vi "MainConvertiMisure_OUTPUT.vi"() -> ()   [LabVIEW 2016]
uses:
  <vilib>/Utility/file.llb/Read Delimited Spreadsheet (string).vi
panel:
  out "Array Miure Convertite":dbl[](array[numeric])
  out "Caratteristiche Caricate":string[][](array[string])
  in  "Array Misure Input":dbl[](array[numeric])
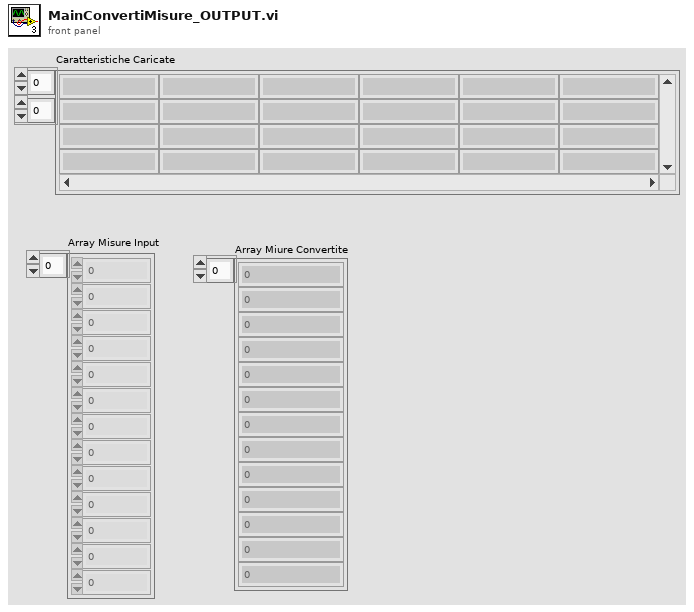
[diagram p1: front panel]
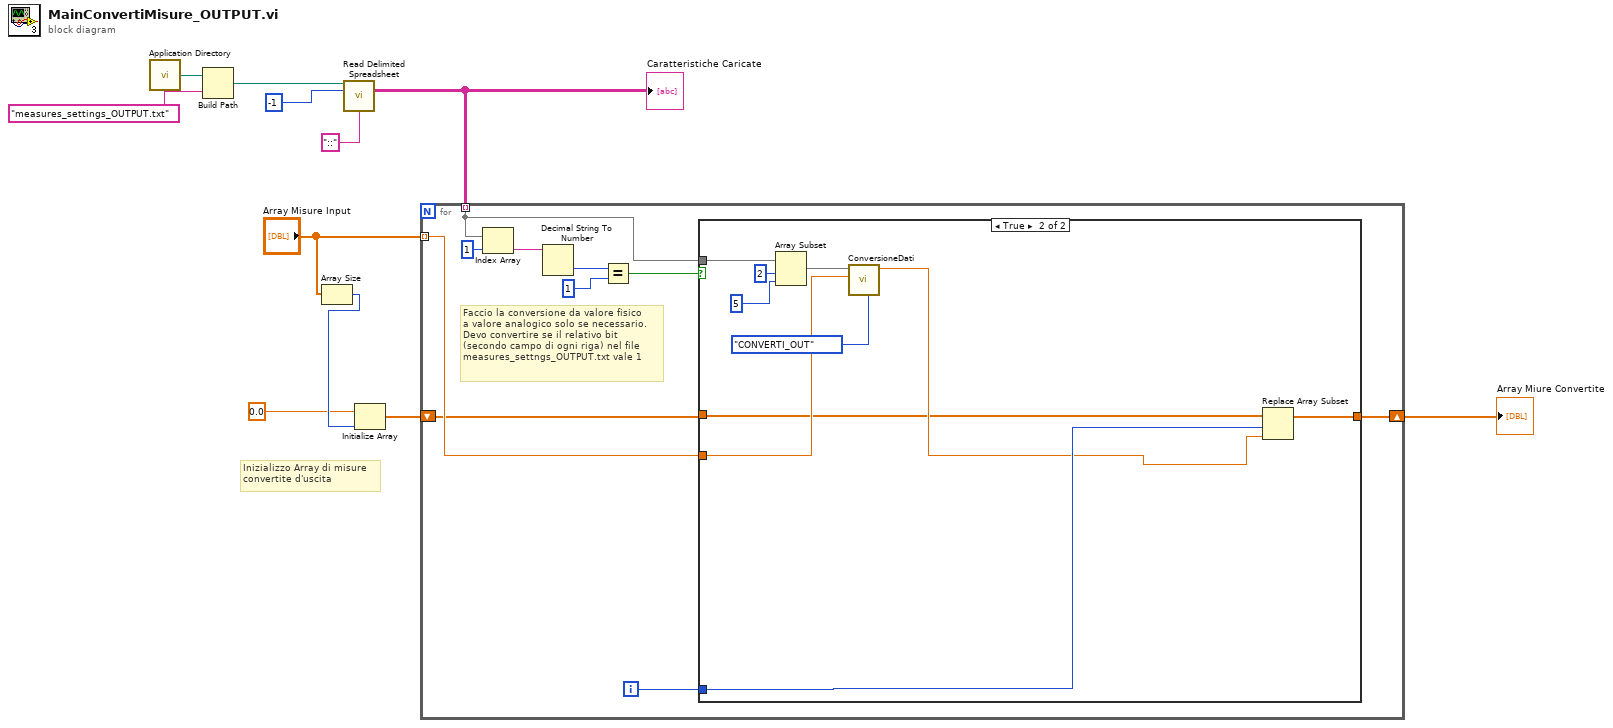
[diagram p0: block diagram]
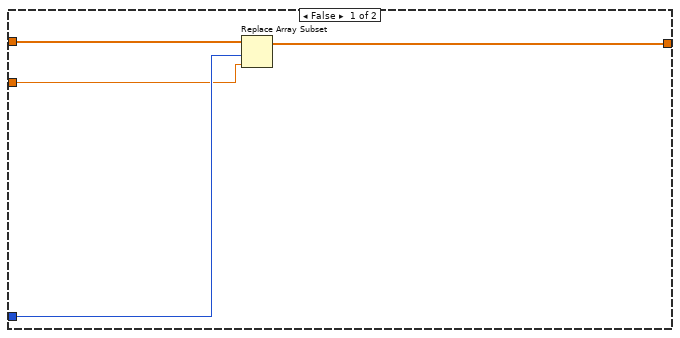
[diagram p2: hidden frame]
diagram:
  # "Inizializzo Array di misure \nconvertite d'uscita"
  n1 = call <vilib>:"Application Directory.vi"() -> ("Application Directory"=w10:path)
  n2 = Build Path(base path=w10, name or relative path="measures_settings_OUTPUT.txt") -> (appended path=w9:path)
  n3 = Array Size(array="Array Misure Input") -> (size(s)=w4:i32)
  n4 = call-poly <vilib>:"Read Delimited Spreadsheet.vi"("file path (dialog if empty)"=w9, "number of rows (all:-1)"=-1, "delimiter (\\t)"="::" ("delimiter (\\t)")) -> ("all rows"=w6:string[][])  [unwired: 7 in, 5 out]
  "Caratteristiche Caricate" <- w6
  n5 = Initialize Array(0.0, w4) -> (w2:dbl[])
  n6 = for {
    tunnel: "Array Misure Input" -> [w16] mode=indexing
    tunnel: w6 -> [w13] mode=indexing
    shift-right: [w14] -> w1
    shift-left: w2 -> [w15]
    i -> [w12]
    # "Faccio la conversione da valore fisico\na valore analogico solo se necessario. \nDevo convertire se il relativo bit \n(secondo campo di ogni riga) nel file \nmeasures_settngs_OUTPUT.txt vale 1"
    n7 = Index Array(array=w13, index=1) -> (element=w20:string)
    n8 = Decimal String To Number(string=w20) -> (number=w19:i32)  [unwired: 2 in, 1 out]
    n9 = Equal?(x=w19, y=1) -> (x = y?=w17:bool)
    n10 = case shown="True" w17 {
      tunnel: w16 -> [w24 w31]
      tunnel: w15 -> [w22 w26]
      tunnel: w12 -> [w25 w35]
      tunnel: [w23 w34] -> w14
      tunnel: w13 -> [_ w33]
      frame False {
        n11 = Replace Array Subset(array=w22, new element=w24, index=w25) -> (w23:dbl[])
      }
      frame True {
        n12 = Array Subset(array=w33, index=2, length=5 ("index")) -> (w32:string[])
        n13 = call "ConversioneDati.vi"("Stato Conversione"=enum16{"CONVERTI_IN", "CONVERTI_OUT"}."CONVERTI_OUT", "Data"=w31, "Impostazioni Conversione"=w32) -> ("Dato Convertito"=w28:dbl)  [unwired: 8 in]
        n14 = Replace Array Subset(array=w26, new element=w28, index=w35) -> (w34:dbl[])
      }
    }
  }
  "Array Miure Convertite" <- w1
